vi "top level batch unzip VI.vi"() -> ()   [LabVIEW 2011]
uses:
  <vilib>/zip/NI_Unzip.lvlib
panel:
  out "Zipping Files":bool
  in  "Zip":bool
  in  "FileType":string caption="File Types (*.CSV)"
  in  "ToZip":path caption="Top Level to scan for files to zip (will scan all sub directories as well)"
  out "UnZipping Files":bool
  out "Scanning":bool
  in  "Zip File Location":T1(ring)
  in  "save unzipped":path caption="Choose a directory to save Unzipped files into."
  in  "Unzipp":bool
  in  "Scan button":bool
  out "Number of Zip files found":i32
  in  "scan dir":path caption="Top Level to scan for *.zip files (will scan all sub directories as well)"
  in  "stop":bool
  # "BATCH UNZIP"
  # "BATCH ZIP"
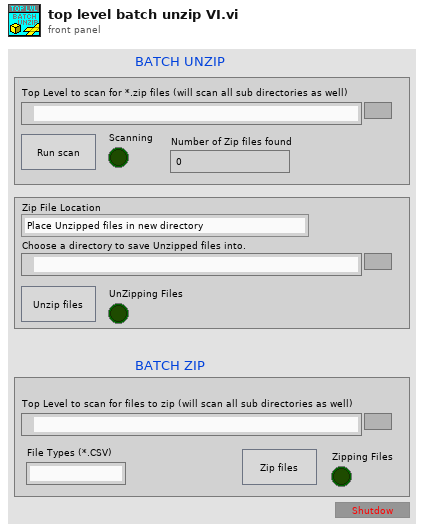
[diagram p1: front panel]
types:
  T1 = enum16{"Place Unzipped files in new directory", "Place Unzipped files in same directory as zip file"}
  T2 = enum8{"Enabled", "Disabled", "Disabled and Grayed Out"}
  T3 = enum32{"invalid app kind", "Development System", "Run Time System", "Student Edition", "Embedded LabVIEW", "Evaluation", "Custom"}
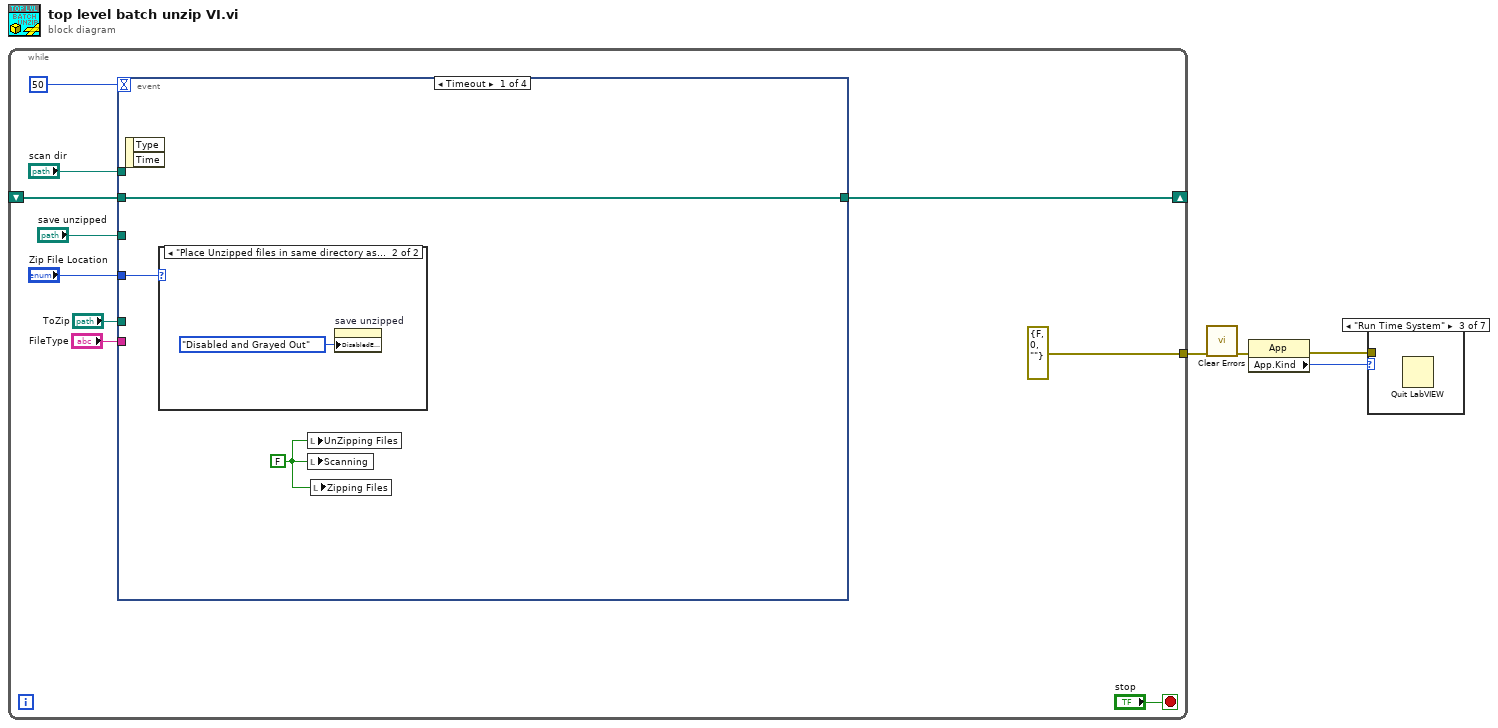
[diagram p0: block diagram]
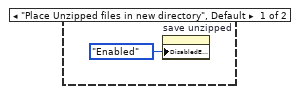
[diagram p8: hidden frame]
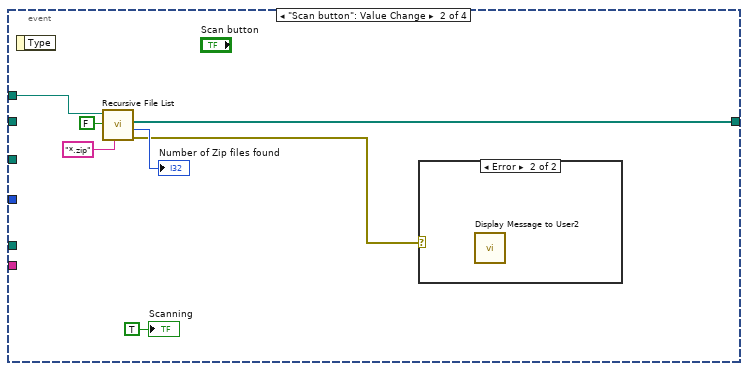
[diagram p9: hidden frame]
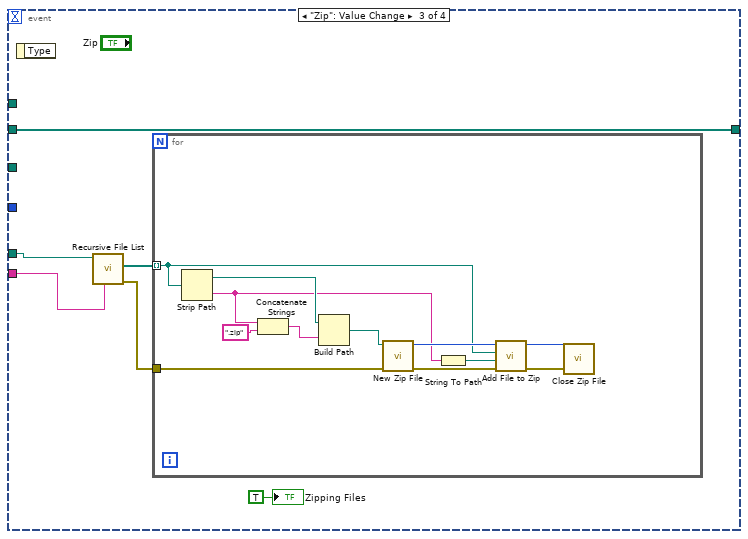
[diagram p11: hidden frame]
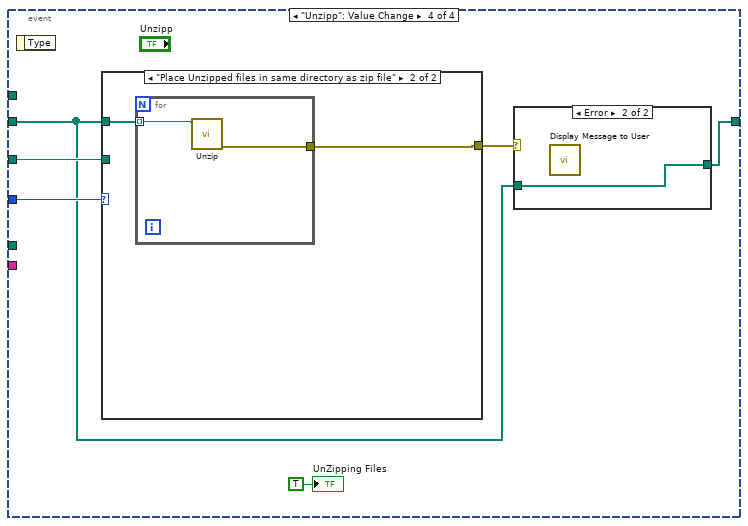
[diagram p12: hidden frame]
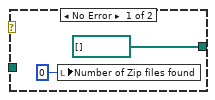
[diagram p13: hidden frame]
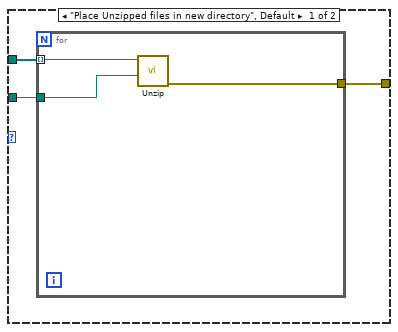
[diagram p14: hidden frame]
diagram:
  n1 = while {
    shift-right: [w12] -> _
    shift-left: _ -> [w11]
    tunnel: [errorcluster {"status"=FALSE, "code"=0, "source"=""} ("error out")] -> w1
    stop <- "stop" stop-if-true
    n2 = event shown="[0] Timeout" {
      selector: _ -> [_ _ _ _]
      dyn-events: _ -> [_ _ _ _]
      timeout: 50 -> [_ _ _ _]
      tunnel: [w16 w23 w28 w47] -> w12
      tunnel: w11 -> [w16 _ w28 w46]
      tunnel: "scan dir" -> [_ w22 _ _]
      tunnel: "Zip File Location" -> [w17 _ _ w50]
      tunnel: "save unzipped" -> [_ _ _ w49]
      tunnel: "ToZip" -> [_ _ w32 _]
      tunnel: "FileType" -> [_ _ w31 _]
      event Timeout {
        w15 = FALSE ("Scanning")
        n3 = event-data() -> ()  [unwired: 1 in, 2 out]
        n4 = case shown="\"Place Unzipped files in same directory as zip file\"" w17 {
          frame "Place Unzipped files in new directory", Default {
            n5 = property on="save unzipped" class="Path"("DisabledEnum"=T2."Enabled" ("Disabled")) -> ()  [unwired: 2 in, 2 out]
          }
          frame "Place Unzipped files in same directory as zip file" {
            n6 = property on="save unzipped" class="Path"("DisabledEnum"=T2."Disabled and Grayed Out" ("Disabled")) -> ()  [unwired: 2 in, 2 out]
          }
        }
        n7 = local write "UnZipping Files"(w15) -> ()
        n8 = local write "Scanning"(w15) -> ()
        n9 = local write "Zipping Files"(w15) -> ()
      }
      event "Scan button": Value Change {
        n10 = event-data() -> ()  [unwired: 1 in, 1 out]
        n11 = call <vilib>:"Recursive File List.vi"("pattern"="*.zip", "Treat LLBs as Folders?"=FALSE, "Folder Path"=w22) -> ("error out"=w21:errorcluster, "Number of Files"=→"Number of Zip files found":i32, "All Files in Dir"=w23:path[])  [unwired: 4 in, 2 out]
        n12 = case shown="Error" w21 {
          frame No Error {
          }
          frame Error {
            n13 = call "Display Message to User2"() -> ()  [unwired: 10 in, 2 out]
          }
        }
        "Scanning" <- TRUE ("Scanning")
      }
      event "Zip": Value Change {
        n14 = event-data() -> ()  [unwired: 1 in, 1 out]
        n15 = call <vilib>:"Recursive File List.vi"("pattern"=w31, "Folder Path"=w32) -> ("error out"=w29:errorcluster, "All Files in Dir"=w30:path[])  [unwired: 5 in, 3 out]
        n16 = for {
          tunnel: w30 -> [w37] mode=indexing
          tunnel: w29 -> [w42]
          n17 = Strip Path(path=w37) -> (stripped path=w36:path, name=w33:string)
          n18 = Concatenate Strings(w33, ".zip" ("string")) -> (w35:string)
          n19 = Build Path(base path=w36, name or relative path=w35) -> (appended path=w34:path)
          n20 = call <vilib>:"New Zip File.vi"("error in (no error)"=w42, "target"=w34) -> ("error out"=w41:errorcluster, "zip file out"=w44:i64)  [unwired: 3 in, 1 out]
          n21 = String To Path(string=w33) -> (path=w38:path)
          n22 = call <vilib>:"Add File to Zip.vi"("error in (no error)"=w41, "destination path in zip"=w38, "source file path"=w37, "zip file in"=w44) -> ("error out"=w40:errorcluster, "zip file out"=w43:i64)  [unwired: 6 in]
          n23 = call <vilib>:"Close Zip File.vi"("error in (no error)"=w40, "zip file in"=w43) -> ()  [unwired: 5 in, 1 out]
        }
        "Zipping Files" <- TRUE ("Zipping Files")
      }
      event "Unzipp": Value Change {
        n24 = event-data() -> ()  [unwired: 1 in, 1 out]
        n25 = case shown="\"Place Unzipped files in same directory as zip file\"" w50 {
          tunnel: w46 -> [w56 w61]
          tunnel: w49 -> [w55 _]
          tunnel: [w54 w60] -> w48
          frame "Place Unzipped files in new directory", Default {
            n26 = for {
              tunnel: w56 -> [w59] mode=indexing
              tunnel: w55 -> [w58]
              tunnel: [w57] -> w54
              n27 = call <vilib>:"Unzip.vi"("Target directory (same as Zip file if empty)"=w58, "Zip file"=w59) -> ("error out"=w57:errorcluster)  [unwired: 7 in, 2 out]
            }
          }
          frame "Place Unzipped files in same directory as zip file" {
            n28 = for {
              tunnel: w61 -> [w63] mode=indexing
              tunnel: [w62] -> w60
              n29 = call <vilib>:"Unzip.vi"("Zip file"=w63) -> ("error out"=w62:errorcluster)  [unwired: 8 in, 2 out]
            }
          }
        }
        n30 = case shown="Error" w48 {
          tunnel: [path[] [] ("All Files in Dir") w53] -> w47
          tunnel: w46 -> [_ w53]
          frame No Error {
            n31 = local write "Number of Zip files found"(0 ("Number of Zip files found")) -> ()
          }
          frame Error {
            n32 = call "Display Message to User"() -> ()  [unwired: 10 in, 2 out]
          }
        }
        "UnZipping Files" <- TRUE ("UnZipping Files")
      }
    }
  }
  n33 = call <vilib>:"Clear Errors.vi"("error in (no error)"=w1) -> ("error out"=w4:errorcluster)  [unwired: 6 in]
  n34 = property class="App"(error in=w4) -> (error out=w3:errorcluster, "App.Kind"=w2:T3)  [unwired: 1 in, 1 out]
  n35 = case shown="\"Run Time System\"" w2 {
    tunnel: w3 -> [_ _ _ _ _ _ _]
    frame "invalid app kind", Default {
    }
    frame "Development System" {
    }
    frame "Run Time System" {
      n36 = Quit LabVIEW() -> ()  [unwired: 1 in]
    }
    frame "Student Edition" {
    }
    frame "Embedded LabVIEW" {
    }
    frame "Evaluation" {
    }
    frame "Custom" {
    }
  }
